vi "_Validate Mass Range.vi"(6 "Run Mode":T1, 7 "Ranges #":i32, 8 "Mass Ranges":T2[](array[typedef]) {"Res" items=["High/High", "Medium/Medium", "Low/Low", "High/Medium", "High/Low", "Medium/High", "Medium/Low", "Low/High", "Low/Medium"]}, 9 "Center/Width":bool) -> (0 "Cycle Time (ms)":dbl, 1 "Current Mass Range":T2={"Start"=50.0, "Stop"=300.0, "Step Size"=0.1, "Steps"=1, "Dwell"=1.0, "Parameters"=[], "Res"=0} {"Res" items=["High/High", "Medium/Medium", "Low/Low", "High/Medium", "High/Low", "Medium/High", "Medium/Low", "Low/High", "Low/Medium"]}, 2 "Mass Ranges Out":T2[](array[typedef]) {"Res" items=["High/High", "Medium/Medium", "Low/Low", "High/Medium", "High/Low", "Medium/High", "Medium/Low", "Low/High", "Low/Medium"]}, 3 "Table out":string[][](array[string]), 4 "Ramp Time (ms)":dbl, 5 "Ranges # Out":i32)   [LabVIEW 2012]
uses:
  Type/_Mass Range Property.ctl
  Type/_Mass Range Parameters.ctl
  Type/_RT Res Type.ctl
  Type/_Run Mode.ctl
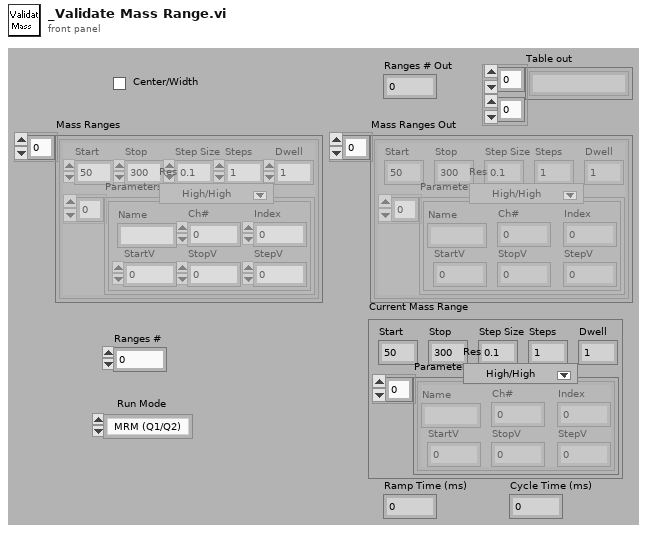
[diagram p1: front panel]
types:
  T1 = typedef "_Run Mode.ctl" = enum16{"MRM (Q1/Q2)", "Q1 Scan", "Q1 SRM", "Q2 Scan", "Q2 SRM", "Product Scan", "Precursor Scan", "Neutral Loss", "Neutral Gain"}
  T2 = typedef "_Mass Range Property.ctl" = cluster{"Start":dbl, "Stop":dbl, "Step Size":dbl, "Steps":i32, "Dwell":dbl, "Parameters":T3[], "Res":T4}
  T3 = typedef "_Mass Range Parameters.ctl" = cluster{"Name":string, "Ch#":u8, "StartV":dbl, "StopV":dbl, "StepV":dbl, "Index":u8}
  T4 = typedef "_RT Res Type.ctl" = u16
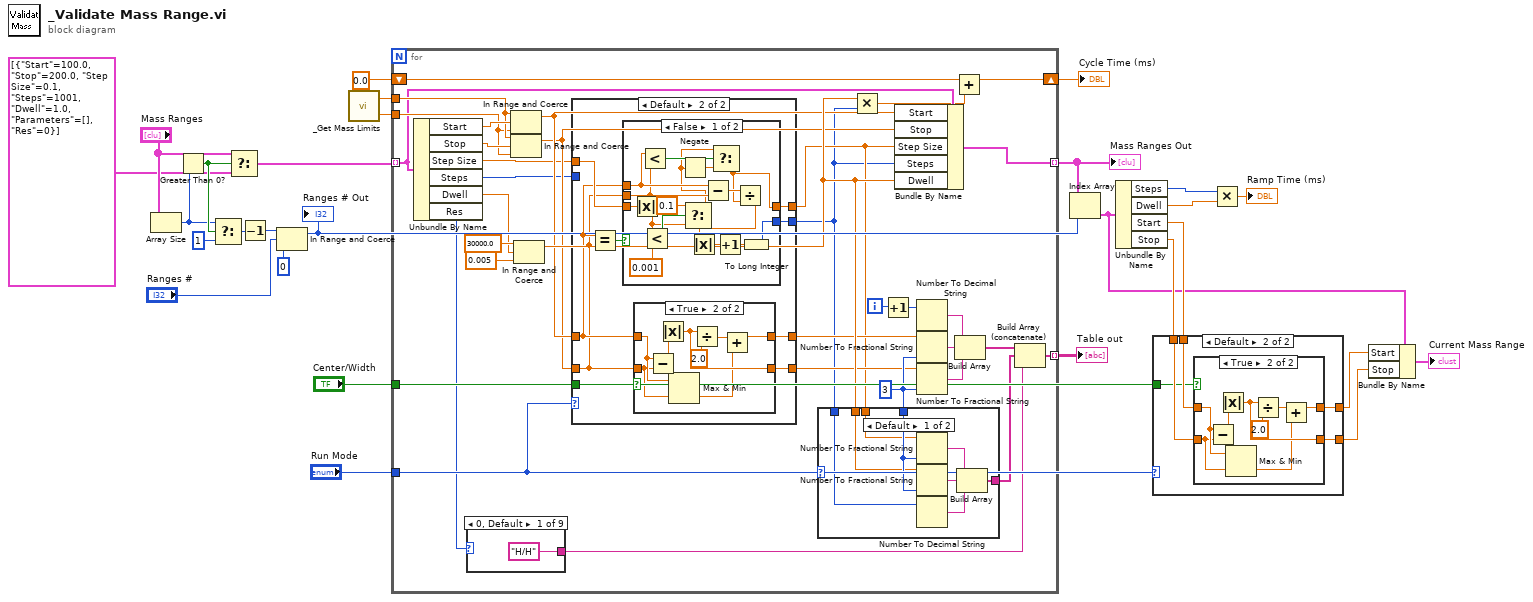
[diagram p0: block diagram]
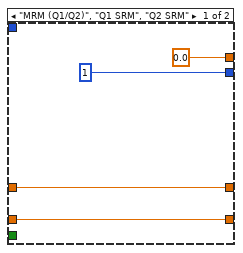
[diagram p4: hidden frame]
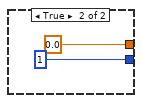
[diagram p5: hidden frame]
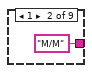
[diagram p7: hidden frame]
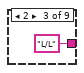
[diagram p8: hidden frame]
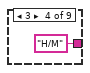
[diagram p9: hidden frame]
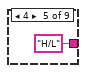
[diagram p10: hidden frame]
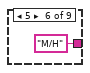
[diagram p11: hidden frame]
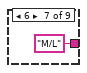
[diagram p12: hidden frame]
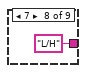
[diagram p13: hidden frame]
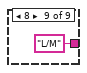
[diagram p14: hidden frame]
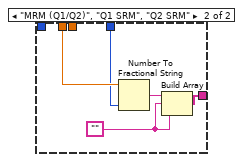
[diagram p15: hidden frame]
diagram:
  n1 = Array Size(array="Mass Ranges") -> (size(s)=w25:i32)
  n2 = Greater Than 0?(x=w25) -> (x > 0?=w26:bool)
  n3 = Select(t=w25, s=w26, f=1) -> (s? t:f=w23:i32)
  n4 = Select(t="Mass Ranges", s=w26, f=T2[] [{"Start"=100.0, "Stop"=200.0, "Step Size"=0.1, "Steps"=1001, "Dwell"=1.0, "Parameters"=[], "Res"=0}] ("Mass Range")) -> (s? t:f=w20:T2[])
  n5 = Decrement(x=w23) -> (x-1=w27:i32)
  n6 = In Range and Coerce(upper limit=w27, x="Ranges #", lower limit=0) -> (coerced(x)=w14:i32)  [unwired: 1 out]
  "Ranges # Out" <- w14
  n7 = call "_Get Mass Limits.vi"() -> ("Max"=w17:dbl, "Min"=w16:dbl)  [unwired: 1 in]
  n8 = for {
    tunnel: w20 -> [w50] mode=indexing
    shift-right: [w47] -> w18
    shift-left: 0.0 -> [w49]
    tunnel: w17 -> [w55]
    tunnel: w16 -> [w54]
    tunnel: [w46] -> w15 mode=indexing
    tunnel: [w41] -> w10 mode=indexing
    tunnel: "Center/Width" -> [w38]
    tunnel: "Run Mode" -> [w29]
    i -> [w62]
    w45 = i16 3 ("precision (6)")
    n9 = Unbundle By Name(w50) -> ("Start"=w57:dbl, "Stop"=w56:dbl, "Step Size"=w31:dbl, "Steps"=w32:i32, "Dwell"=w51:dbl, "Res"=w40:T4)
    n10 = case shown="0, Default" w40 {
      tunnel: ["H/H" "M/M" "L/L" "H/M" "H/L" "M/H" "M/L" "L/H" "L/M"] -> w39
      frame 0, Default {
      }
      frame 1 {
      }
      frame 2 {
      }
      frame 3 {
      }
      frame 4 {
      }
      frame 5 {
      }
      frame 6 {
      }
      frame 7 {
      }
      frame 8 {
      }
    }
    n11 = In Range and Coerce(upper limit=w55, x=w57, lower limit=w54) -> (coerced(x)=w37:dbl)  [unwired: 1 out]
    n12 = In Range and Coerce(upper limit=w55, x=w56, lower limit=w54) -> (coerced(x)=w36:dbl)  [unwired: 1 out]
    n13 = In Range and Coerce(upper limit=30000.0, x=w51, lower limit=0.005) -> (coerced(x)=w44:dbl)  [unwired: 1 out]
    n14 = case shown="Default" w29 {
      tunnel: w37 -> [w66 w69]
      tunnel: w36 -> [w65 w68]
      tunnel: [w66 w75] -> w35
      tunnel: [w65 w74] -> w34
      tunnel: w38 -> [_ w73]
      tunnel: [1 ("Steps") w71] -> w30
      tunnel: [0.0 w72] -> w33
      tunnel: w32 -> [_ _]
      tunnel: w31 -> [_ w70]
      frame "MRM (Q1/Q2)", "Q1 SRM", "Q2 SRM" {
      }
      frame Default {
        n15 = Equal?(x=w69, y=w68) -> (x = y?=w67:bool)
        n16 = case shown="False" w67 {
          tunnel: w69 -> [w87 _]
          tunnel: [w83 1 ("Steps")] -> w71
          tunnel: w68 -> [w86 _]
          tunnel: [w85 0.0] -> w72
          tunnel: w70 -> [w90 _]
          frame False {
            n17 = Absolute Value(x=w90) -> (abs(x)=w77:dbl)
            n18 = Less?(x=w87, y=w86) -> (x < y?=w89:bool)
            n19 = Less?(x=w77, y=0.001) -> (x < y?=w78:bool)
            n20 = Select(t=0.1, s=w78, f=w77) -> (s? t:f=w76:dbl)
            n21 = Negate(x=w76) -> (-x=w88:dbl)
            n22 = Subtract(x=w87, y=w86) -> (x-y=w91:dbl)
            n23 = Select(t=w76, s=w89, f=w88) -> (s? t:f=w85:dbl)
            n24 = Divide(x=w91, y=w85) -> (x/y=w81:dbl)
            n25 = Absolute Value(x=w81) -> (abs(x)=w84:dbl)
            n26 = Increment(x=w84) -> (x+1=w82:dbl)
            n27 = To Long Integer(number=w82) -> (32bit integer=w83:i32)
          }
          frame True {
          }
        }
        n28 = case shown="True" w73 {
          tunnel: w69 -> [w95 w99]
          tunnel: w68 -> [w94 w98]
          tunnel: [w95 w96] -> w75
          tunnel: [w94 w101] -> w74
          frame False {
          }
          frame True {
            n29 = Subtract(x=w99, y=w98) -> (x-y=w102:dbl)
            n30 = Absolute Value(x=w102) -> (abs(x)=w101:dbl)
            n31 = Max & Min(x=w99, y=w98) -> (min(x,y)=w97:dbl)  [unwired: 1 out]
            n32 = Divide(x=w101, y=2.0) -> (x/y=w100:dbl)
            n33 = Add(x=w100, y=w97) -> (x+y=w96:dbl)
          }
        }
      }
    }
    n34 = case shown="Default" w29 {
      tunnel: w45 -> [w120 w122]
      tunnel: w33 -> [w119 _]
      tunnel: w44 -> [w118 w125]
      tunnel: w30 -> [w113 _]
      tunnel: [w114 w123] -> w42
      frame Default {
        n35 = Number To Fractional String(number=w119, precision (6)=w120) -> (F-format string=w117:string)  [unwired: 2 out]
        n36 = Number To Fractional String(number=w118, precision (6)=w120) -> (F-format string=w115:string)  [unwired: 2 out]
        n37 = Number To Decimal String(number=w113) -> (decimal integer string=w116:string)  [unwired: 1 out]
        n38 = Build Array(w117, w115, w116) -> (w114:string[])
      }
      frame "MRM (Q1/Q2)", "Q1 SRM", "Q2 SRM" {
        w121 = ""
        n39 = Number To Fractional String(number=w125, precision (6)=w122) -> (F-format string=w124:string)  [unwired: 2 out]
        n40 = Build Array(w124, w121, w121) -> (w123:string[])
      }
    }
    n41 = Multiply(x=w44, y=w30) -> (x*y=w48:dbl)
    n42 = Increment(x=w62) -> (x+1=w61:i32)
    n43 = Bundle By Name(cluster=w50, "Start"=w37, "Stop"=w36, "Step Size"=w33, "Steps"=w30, "Dwell"=w44) -> (w46:T2)
    n44 = Number To Decimal String(number=w61) -> (decimal integer string=w60:string)  [unwired: 1 out]
    n45 = Number To Fractional String(number=w35, precision (6)=w45) -> (F-format string=w59:string)  [unwired: 2 out]
    n46 = Number To Fractional String(number=w34, precision (6)=w45) -> (F-format string=w58:string)  [unwired: 2 out]
    n47 = Add(x=w49, y=w48) -> (x+y=w47:dbl)
    n48 = Build Array(w60, w59, w58) -> (w43:string[])
    n49 = Build Array (concatenate)(w43, w42, w39) -> (w41:string[])
  }
  "Table out" <- w10
  "Cycle Time (ms)" <- w18
  "Mass Ranges Out" <- w15
  n50 = Index Array(array=w15, index=w14) -> (element=w5:T2)
  n51 = Unbundle By Name(w5) -> ("Steps"=w13:i32, "Dwell"=w12:dbl, "Start"=w7:dbl, "Stop"=w6:dbl)
  n52 = case shown="Default" "Run Mode" {
    tunnel: [w127 w132] -> w4
    tunnel: [w126 w131] -> w3
    tunnel: "Center/Width" -> [_ w128]
    tunnel: w7 -> [w127 w130]
    tunnel: w6 -> [w126 w129]
    frame "MRM (Q1/Q2)", "Q1 SRM", "Q2 SRM" {
    }
    frame Default {
      n53 = case shown="True" w128 {
        tunnel: w130 -> [w134 w137]
        tunnel: w129 -> [w133 w136]
        tunnel: [w134 w138] -> w132
        tunnel: [w133 w140] -> w131
        frame False {
        }
        frame True {
          n54 = Subtract(x=w137, y=w136) -> (x-y=w141:dbl)
          n55 = Absolute Value(x=w141) -> (abs(x)=w140:dbl)
          n56 = Max & Min(x=w137, y=w136) -> (min(x,y)=w135:dbl)  [unwired: 1 out]
          n57 = Divide(x=w140, y=2.0) -> (x/y=w139:dbl)
          n58 = Add(x=w139, y=w135) -> (x+y=w138:dbl)
        }
      }
    }
  }
  n59 = Multiply(x=w13, y=w12) -> (x*y=→"Ramp Time (ms)":dbl)
  n60 = Bundle By Name(cluster=w5, "Start"=w4, "Stop"=w3) -> (→"Current Mass Range":T2)
